vi "DataLogger_SetFileRef.vi"(8 "error in (no error)":errorcluster, 10 "File reference":refnum<file>, 11 "Data Logger in":refnum<class "Data Logger.lvclass">) -> (0 "error out":errorcluster, 3 "Data Logger out":refnum<class "Data Logger.lvclass">)   [LabVIEW 2015, in "Data Logger.lvclass"]
uses:
  Data Logger.lvclass
  Data Logger.lvclass/Data Logger.ctl
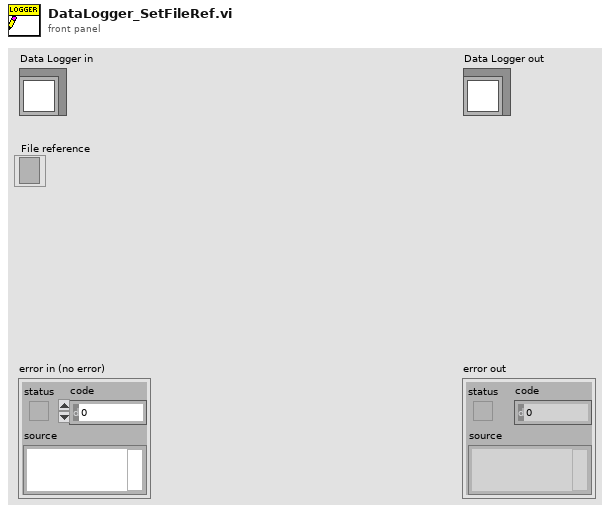
[diagram p1: front panel]
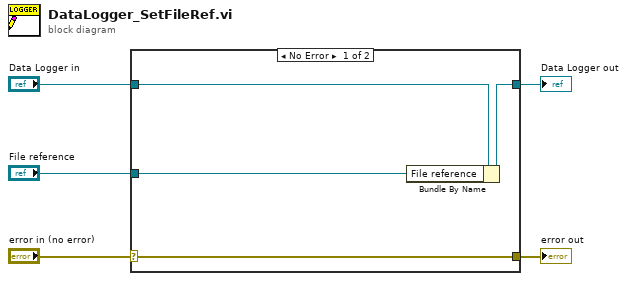
[diagram p0: block diagram]
diagram:
  n1 = case shown="No Error" "error in (no error)" {
    selector: "error in (no error)" -> [w9 w10]
    tunnel: [w9 w10] -> w4
    tunnel: [w7 w11] -> w2
    tunnel: "Data Logger in" -> [w8 w11]
    tunnel: "File reference" -> [w6 _]
    frame No Error {
      n2 = Bundle By Name(cluster=w8, "File reference"=w6) -> (w7:refnum<class "Data Logger.lvclass">)
    }
    frame Error {
    }
  }
  "error out" <- w4
  "Data Logger out" <- w2
